vi "moments_of_p(u_v)_m.vi"(8 "constants":T1={"u'/U"=0.5, "v'/U"=0.4, "w'/U"=0.4, "rho"=0.5, "alpha1"=0.0, "alpha2"=0.0} {"alpha2" format="%.2f"; "alpha1" format="%.2f"; "rho" format="%.2f"; "w'/U" format="%.2f"; "v'/U" format="%.2f"; "u'/U" format="%.2f"}, 9 "u*, v* limits":T2={"u* low"=0.4, "u* high"=1.8, "v* low"=-0.6, "v* high"=0.8} {"v* high" format="%.2f"; "v* low" format="%.2f"; "u* high" format="%.2f"; "u* low" format="%.2f"}, 10 "grid size for z*":i16=16, 11 "grid size for u* and v*":i16=32) -> (1 "Results table":string[][](table), 3 "Volume under p(u*,v*)":dbl format="%.5f")   [LabVIEW 2010]
uses:
  <vilib>/Analysis/NI_AALPro.lvlib
panel:
  out "run time (s)":u32
  out "v*^2":dbl format="%.5f"
  out "u*^2":dbl format="%.5f"
  out "plot 2":dbl[][](graph)
  out "V*":dbl format="%.5f"
  out "plot 1":dbl[][](graph)
  out "U*":dbl format="%.5f"
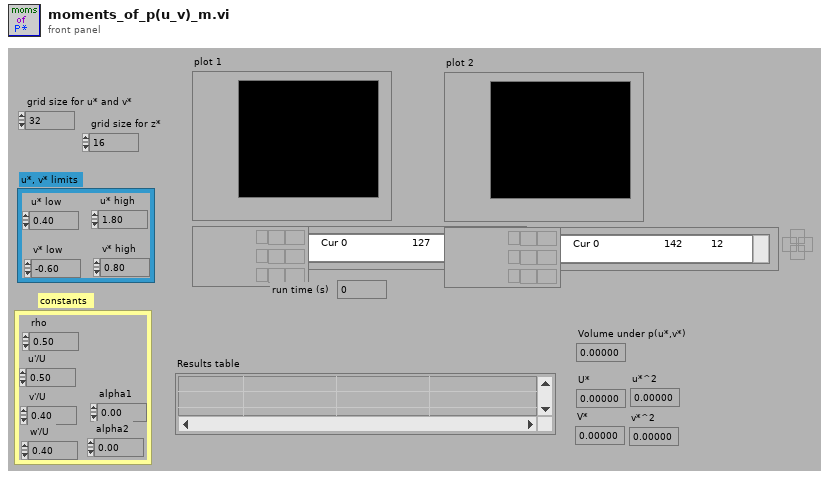
[diagram p1: front panel]
types:
  T1 = cluster{"u'/U":dbl, "v'/U":dbl, "w'/U":dbl, "rho":dbl, "alpha1":dbl, "alpha2":dbl}
  T2 = cluster{"u* low":dbl, "u* high":dbl, "v* low":dbl, "v* high":dbl}
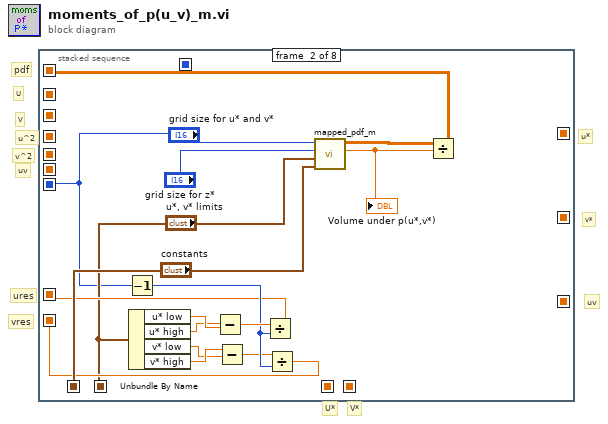
[diagram p0: block diagram]
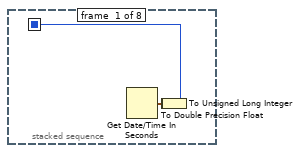
[diagram p2: hidden frame]
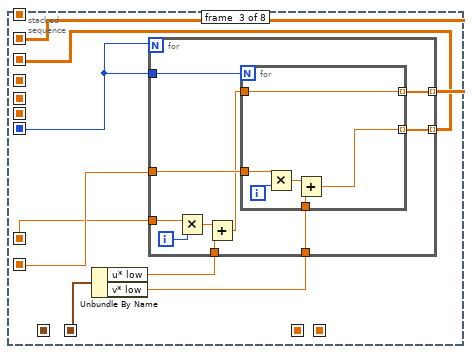
[diagram p3: hidden frame]
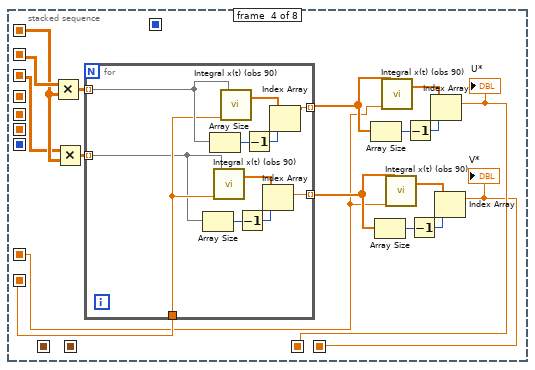
[diagram p4: hidden frame]
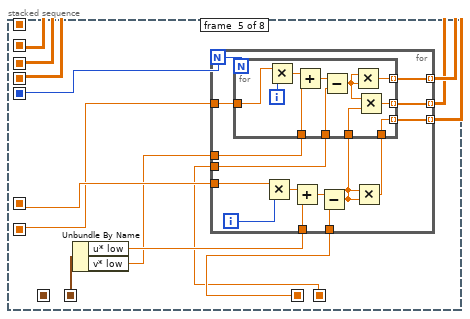
[diagram p5: hidden frame]
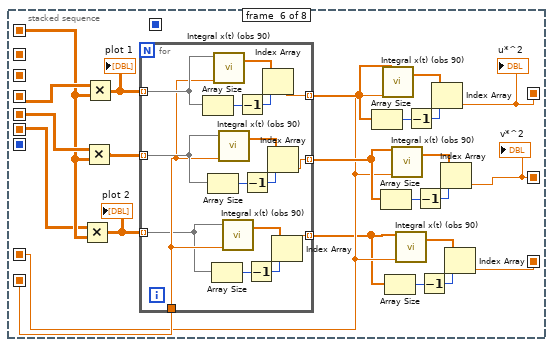
[diagram p6: hidden frame]
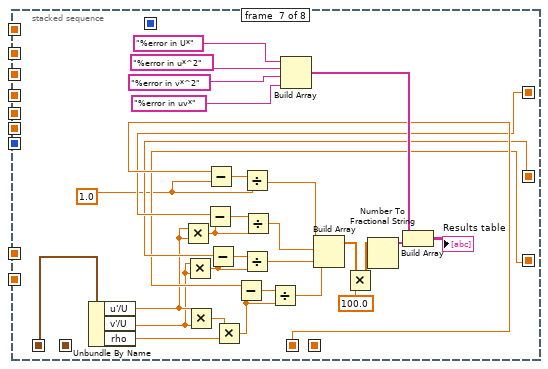
[diagram p7: hidden frame]
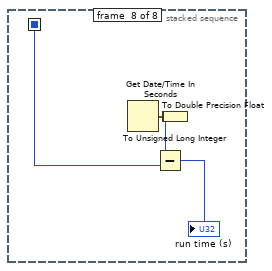
[diagram p8: hidden frame]
diagram:
  # "uv"
  # "uv"
  # "v*"
  # "u*"
  # "V*"
  # "U*"
  # "V"
  # "v^2"
  # "u^2"
  # "U"
  # "pdf"
  # "vres"
  # "ures"
  n1 = stacked-sequence {
    seq-local: [_ w6 _ _ _ _ _ _] -> [_ _ _ w53 _ w117 _ _]
    seq-local: [_ w9 _ _ _ _ _ _] -> [_ _ w22 w46 w82 w118 _ _]
    seq-local: [_ w8 _ _ _ _ _ _] -> [_ _ w23 w60 w77 w132 _ _]
    seq-local: [_ "u*, v* limits" _ _ _ _ _ _] -> [_ _ w27 _ w81 _ _ _]
    seq-local: [_ _ w21 _ _ _ _ _] -> [_ _ _ w55 _ _ _ _]
    seq-local: [_ "grid size for u* and v*" _ _ _ _ _ _] -> [_ _ w26 _ w73 _ _ _]
    seq-local: [_ "constants" _ _ _ _ _ _] -> [_ _ _ _ _ _ w176 _]
    seq-local: [_ _ _ _ w74 _ _ _] -> [_ _ _ _ _ w129 _ _]
    seq-local: [_ _ _ _ w75 _ _ _] -> [_ _ _ _ _ w128 _ _]
    seq-local: [_ _ _ _ _ w109 _ _] -> [_ _ _ _ _ _ w165 _]
    seq-local: [_ _ _ _ _ w110 _ _] -> [_ _ _ _ _ _ w164 _]
    seq-local: [_ _ w20 _ _ _ _ _] -> [_ _ _ w47 _ _ _ _]
    seq-local: [_ _ _ w45 _ _ _ _] -> [_ _ _ _ w79 _ w166 _]
    seq-local: [_ _ _ w44 _ _ _ _] -> [_ _ _ _ w76 _ _ _]
    seq-local: [_ _ _ _ w72 _ _ _] -> [_ _ _ _ _ w116 _ _]
    seq-local: [_ _ _ _ _ w114 _ _] -> [_ _ _ _ _ _ w154 _]
    seq-local: [w3 _ _ _ _ _ _ _] -> [_ _ _ _ _ _ _ w183]
    frame #0 {
      n2 = Get Date/Time In Seconds() -> (seconds since 1Jan1904=w1:timestamp)
      n3 = To Double Precision Float(number=w1) -> (double precision float=w2:dbl)
      n4 = To Unsigned Long Integer(number=w2) -> (unsigned 32bit integer=w3:u32)
    }
    frame #1 {
      n5 = Decrement(x="grid size for u* and v*") -> (x-1=w11:i16)
      n6 = Unbundle By Name("u*, v* limits") -> ("u* low"=w16:dbl, "u* high"=w15:dbl, "v* low"=w13:dbl, "v* high"=w14:dbl)
      n7 = Subtract(x=w15, y=w16) -> (x-y=w12:dbl)
      n8 = Subtract(x=w14, y=w13) -> (x-y=w10:dbl)
      n9 = Divide(x=w12, y=w11) -> (x/y=w9:dbl)
      n10 = Divide(x=w10, y=w11) -> (x/y=w8:dbl)
      n11 = call "mapped_pdf_m.vi"("constants"="constants", "u*, v* limits"="u*, v* limits", "grid size for z*"="grid size for z*", "grid size for u* and v*"="grid size for u* and v*") -> ("Volume under p(u*,v*)"=w18:dbl, "p(u*,v*)"=w7:dbl[][])  [unwired: 4 out]
      "Volume under p(u*,v*)" <- w18
      n12 = Divide(x=w7, y=w18) -> (x/y=w6:dbl[][])
    }
    frame #2 {
      n13 = Unbundle By Name(w27) -> ("u* low"=w25:dbl, "v* low"=w24:dbl)
      n14 = for {
        N: w26 -> [_]
        tunnel: w22 -> [w37]
        tunnel: w23 -> [w36]
        tunnel: w26 -> [w33]
        tunnel: w25 -> [w32]
        tunnel: w24 -> [w31]
        tunnel: [w30] -> w21 mode=indexing
        tunnel: [w28] -> w20 mode=indexing
        i -> [w34]
        n15 = Multiply(x=w37, y=w34) -> (x*y=w35:dbl)
        n16 = Add(x=w35, y=w32) -> (x+y=w29:dbl)
        n17 = for {
          N: w33 -> [_]
          tunnel: w36 -> [w41]
          tunnel: w31 -> [w40]
          tunnel: [w39] -> w30 mode=indexing
          tunnel: w29 -> [w39]
          tunnel: [w38] -> w28 mode=indexing
          i -> [w42]
          n18 = Multiply(x=w41, y=w42) -> (x*y=w43:dbl)
          n19 = Add(x=w43, y=w40) -> (x+y=w38:dbl)
        }
      }
    }
    frame #3 {
      n20 = Multiply(x=w55, y=w53) -> (x*y=w54:dbl[][])
      n21 = Multiply(x=w47, y=w53) -> (x*y=w48:dbl[][])
      n22 = for {
        tunnel: w60 -> [w63]
        tunnel: [w68] -> w56 mode=indexing
        tunnel: w54 -> [w64] mode=indexing
        tunnel: w48 -> [w62] mode=indexing
        tunnel: [w61] -> w49 mode=indexing
        n23 = Array Size(array=w62) -> (size(s)=w70:i32)
        n24 = Array Size(array=w64) -> (size(s)=w66:i32)
        n25 = call <vilib>:"Integral x(t) (obs 90).vi"("dt"=w63, "X"=w62) -> ("Integral X"=w71:dbl[])  [unwired: 2 in, 1 out]
        n26 = call <vilib>:"Integral x(t) (obs 90).vi"("dt"=w63, "X"=w64) -> ("Integral X"=w65:dbl[])  [unwired: 2 in, 1 out]
        n27 = Decrement(x=w70) -> (x-1=w69:i32)
        n28 = Decrement(x=w66) -> (x-1=w67:i32)
        n29 = Index Array(array=w71, index=w69) -> (element=w68:dbl)
        n30 = Index Array(array=w65, index=w67) -> (element=w61:dbl)
      }
      n31 = Array Size(array=w49) -> (size(s)=w51:i32)
      n32 = Array Size(array=w56) -> (size(s)=w58:i32)
      n33 = call <vilib>:"Integral x(t) (obs 90).vi"("dt"=w46, "X"=w49) -> ("Integral X"=w52:dbl[])  [unwired: 2 in, 1 out]
      n34 = call <vilib>:"Integral x(t) (obs 90).vi"("dt"=w46, "X"=w56) -> ("Integral X"=w57:dbl[])  [unwired: 2 in, 1 out]
      n35 = Decrement(x=w51) -> (x-1=w50:i32)
      n36 = Decrement(x=w58) -> (x-1=w59:i32)
      n37 = Index Array(array=w52, index=w50) -> (element=w45:dbl)
      "U*" <- w45
      n38 = Index Array(array=w57, index=w59) -> (element=w44:dbl)
      "V*" <- w44
    }
    frame #4 {
      n39 = Unbundle By Name(w81) -> ("u* low"=w80:dbl, "v* low"=w78:dbl)
      n40 = for {
        N: w73 -> [w85]
        tunnel: w82 -> [w96]
        tunnel: w80 -> [w94]
        tunnel: w79 -> [w92]
        tunnel: w78 -> [w91]
        tunnel: w77 -> [w90]
        tunnel: w76 -> [w89]
        tunnel: [w87] -> w74 mode=indexing
        tunnel: [w86] -> w75 mode=indexing
        tunnel: [w83] -> w72 mode=indexing
        i -> [w97]
        n41 = Multiply(x=w96, y=w97) -> (x*y=w95:dbl)
        n42 = Add(x=w95, y=w94) -> (x+y=w93:dbl)
        n43 = Subtract(x=w93, y=w92) -> (x-y=w84:dbl)
        n44 = Multiply(x=w84, y=w84) -> (x*y=w88:dbl)
        n45 = for {
          N: w85 -> [_]
          tunnel: w91 -> [w106]
          tunnel: w90 -> [w105]
          tunnel: w89 -> [w103]
          tunnel: [w102] -> w86 mode=indexing
          tunnel: [w101] -> w87 mode=indexing
          tunnel: w88 -> [w101]
          tunnel: w84 -> [w99]
          tunnel: [w98] -> w83 mode=indexing
          i -> [w104]
          n46 = Multiply(x=w105, y=w104) -> (x*y=w107:dbl)
          n47 = Add(x=w107, y=w106) -> (x+y=w108:dbl)
          n48 = Subtract(x=w108, y=w103) -> (x-y=w100:dbl)
          n49 = Multiply(x=w100, y=w100) -> (x*y=w102:dbl)
          n50 = Multiply(x=w100, y=w99) -> (x*y=w98:dbl)
        }
      }
    }
    frame #5 {
      n51 = Multiply(x=w116, y=w117) -> (x*y=w111:dbl[][])
      "plot 2" <- w111
      n52 = Multiply(x=w128, y=w117) -> (x*y=w113:dbl[][])
      n53 = Multiply(x=w129, y=w117) -> (x*y=w112:dbl[][])
      "plot 1" <- w112
      n54 = for {
        tunnel: w132 -> [w135]
        tunnel: [w145] -> w122 mode=indexing
        tunnel: w113 -> [w140] mode=indexing
        tunnel: w112 -> [w141] mode=indexing
        tunnel: [w139] -> w124 mode=indexing
        tunnel: w111 -> [w134] mode=indexing
        tunnel: [w133] -> w115 mode=indexing
        n55 = Array Size(array=w141) -> (size(s)=w147:i32)
        n56 = Array Size(array=w140) -> (size(s)=w143:i32)
        n57 = Array Size(array=w134) -> (size(s)=w137:i32)
        n58 = call <vilib>:"Integral x(t) (obs 90).vi"("dt"=w135, "X"=w141) -> ("Integral X"=w148:dbl[])  [unwired: 2 in, 1 out]
        n59 = call <vilib>:"Integral x(t) (obs 90).vi"("dt"=w135, "X"=w140) -> ("Integral X"=w144:dbl[])  [unwired: 2 in, 1 out]
        n60 = call <vilib>:"Integral x(t) (obs 90).vi"("dt"=w135, "X"=w134) -> ("Integral X"=w136:dbl[])  [unwired: 2 in, 1 out]
        n61 = Decrement(x=w147) -> (x-1=w146:i32)
        n62 = Decrement(x=w143) -> (x-1=w142:i32)
        n63 = Decrement(x=w137) -> (x-1=w138:i32)
        n64 = Index Array(array=w148, index=w146) -> (element=w145:dbl)
        n65 = Index Array(array=w144, index=w142) -> (element=w139:dbl)
        n66 = Index Array(array=w136, index=w138) -> (element=w133:dbl)
      }
      n67 = Array Size(array=w122) -> (size(s)=w130:i32)
      n68 = Array Size(array=w124) -> (size(s)=w126:i32)
      n69 = call <vilib>:"Integral x(t) (obs 90).vi"("dt"=w118, "X"=w122) -> ("Integral X"=w123:dbl[])  [unwired: 2 in, 1 out]
      n70 = Array Size(array=w115) -> (size(s)=w120:i32)
      n71 = call <vilib>:"Integral x(t) (obs 90).vi"("dt"=w118, "X"=w124) -> ("Integral X"=w127:dbl[])  [unwired: 2 in, 1 out]
      n72 = call <vilib>:"Integral x(t) (obs 90).vi"("dt"=w118, "X"=w115) -> ("Integral X"=w119:dbl[])  [unwired: 2 in, 1 out]
      n73 = Decrement(x=w130) -> (x-1=w131:i32)
      n74 = Decrement(x=w126) -> (x-1=w125:i32)
      n75 = Decrement(x=w120) -> (x-1=w121:i32)
      n76 = Index Array(array=w123, index=w131) -> (element=w109:dbl)
      "u*^2" <- w109
      n77 = Index Array(array=w127, index=w125) -> (element=w110:dbl)
      "v*^2" <- w110
      n78 = Index Array(array=w119, index=w121) -> (element=w114:dbl)
    }
    frame #6 {
      w149 = 1.0
      n79 = Unbundle By Name(w176) -> ("u'/U"=w153:dbl, "v'/U"=w150:dbl, "rho"=w161:dbl)
      n80 = Multiply(x=w153, y=w153) -> (x*y=w152:dbl)
      n81 = Multiply(x=w150, y=w150) -> (x*y=w151:dbl)
      n82 = Multiply(x=w153, y=w150) -> (x*y=w162:dbl)
      n83 = Subtract(x=w165, y=w152) -> (x-y=w171:dbl)
      n84 = Subtract(x=w166, y=w149) -> (x-y=w170:dbl)
      n85 = Subtract(x=w164, y=w151) -> (x-y=w172:dbl)
      n86 = Multiply(x=w162, y=w161) -> (x*y=w159:dbl)
      n87 = Subtract(x=w154, y=w159) -> (x-y=w160:dbl)
      n88 = Divide(x=w170, y=w149) -> (x/y=w167:dbl)
      n89 = Divide(x=w172, y=w151) -> (x/y=w169:dbl)
      n90 = Divide(x=w171, y=w152) -> (x/y=w168:dbl)
      n91 = Divide(x=w160, y=w159) -> (x/y=w158:dbl)
      n92 = Build Array("%error in U*", "%error in u*^2", "%error in v*^2", "%error in uv*") -> (w174:string[])
      n93 = Build Array(w167, w168, w169, w158) -> (w156:dbl[])
      n94 = Multiply(x=w156, y=100.0) -> (x*y=w155:dbl[])
      n95 = Number To Fractional String(number=w155) -> (F-format string=w175:string[])  [unwired: 3 out]
      n96 = Build Array(w174, w175) -> (→"Results table":string[][])
    }
    frame #7 {
      n97 = Get Date/Time In Seconds() -> (seconds since 1Jan1904=w180:timestamp)
      n98 = To Double Precision Float(number=w180) -> (double precision float=w181:dbl)
      n99 = To Unsigned Long Integer(number=w181) -> (unsigned 32bit integer=w184:u32)
      n100 = Subtract(x=w184, y=w183) -> (x-y=→"run time (s)":u32)
    }
  }
